vi "MakeHeaderFile.vi"(4 "Data File Name 2":path, 5 "Data File Name 1":path, 6 "Parameters":string, 7 "File Format":T1, 8 "error in (no error)":errorcluster, 9 "File Description":string, 10 "File Name":path, 11 "Date/Time sec (Now if empty)":dbl format="%.2f") -> (0 "error out":errorcluster, 1 "Complete text":string, 3 "Actual date/time":string)   [LabVIEW 2015]
uses:
  Controls/File formats.ctl
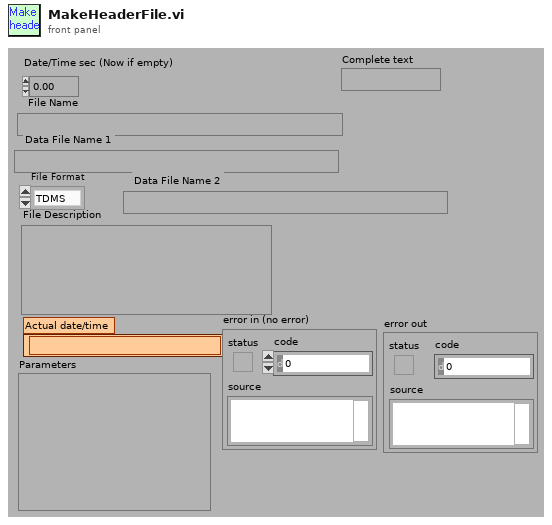
[diagram p1: front panel]
types:
  T1 = typedef "File formats.ctl" = enum16{"TDMS", "ASCII", "BINARY"}
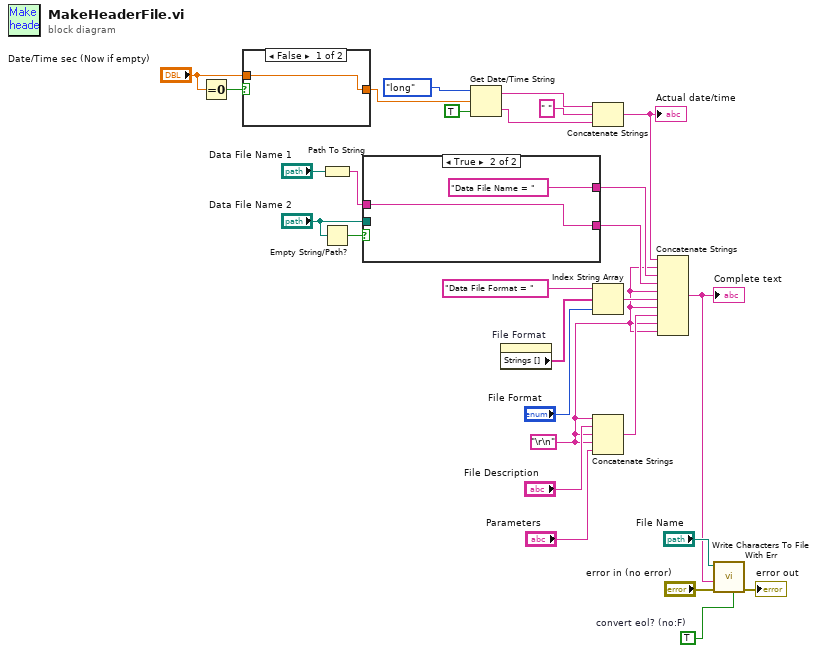
[diagram p0: block diagram]
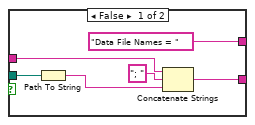
[diagram p2: hidden frame]
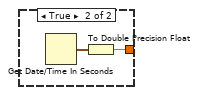
[diagram p3: hidden frame]
diagram:
  w25 = TRUE  # convert eol? (no:F)
  w3 = "\r\n"
  n1 = Equal To 0?(x="Date/Time sec (Now if empty)") -> (x = 0?=w18:bool)
  n2 = case shown="False" w18 {
    tunnel: [w29 w31] -> w24
    tunnel: "Date/Time sec (Now if empty)" -> [w29 _]
    frame False {
    }
    frame True {
      n3 = Get Date/Time In Seconds() -> (seconds since 1Jan1904=w30:timestamp)
      n4 = To Double Precision Float(number=w30) -> (double precision float=w31:dbl)
    }
  }
  n5 = Path To String(path="Data File Name 1") -> (string=w9:string)
  n6 = Empty String/Path?(string/path="Data File Name 2") -> (empty?=w8:bool)
  n7 = case shown="True" w8 {
    tunnel: w9 -> [w37 w39]
    tunnel: "Data File Name 2" -> [w36 _]
    tunnel: [w33 w39] -> w5
    tunnel: ["Data File Names = " ("Substring") "Data File Name = " ("Substring")] -> w6
    frame False {
      n8 = Path To String(path=w36) -> (string=w35:string)
      n9 = Concatenate Strings(w37, "; " ("Substring"), w35) -> (w33:string)
    }
    frame True {
    }
  }
  n10 = Get Date/Time String(date format (0)=enum16{"short", "long", "abbreviated"}."long", seconds (now)=w24, want seconds? (F)=TRUE) -> (date string=w22:string, time string=w21:string)
  n11 = property on="File Format" class="Enum (strict)"() -> ("Strings []"=w13:string[])  [unwired: 2 in, 2 out]
  n12 = Concatenate Strings(w22, " " ("time string"), w21) -> (w10:string)
  "Actual date/time" <- w10
  n13 = Index String Array(1:"File Format", 2:w13, 3:"Data File Format = " ("string (\"\")")) -> (0:w4:string)
  n14 = Concatenate Strings(w3, "File Description", w3, w3, "Parameters") -> (w26:string)
  n15 = Concatenate Strings(w10, w3, w6, w5, w3, w4, w3, w26, w3, w3) -> (w27:string)
  "Complete text" <- w27
  n16 = call "Write Characters To File With Err.vi"("convert eol? (no:F)"=w25, "error in (no error)"="error in (no error)", "character string"=w27, "file path (dialog if empty)"="File Name") -> ("error out"=→"error out":errorcluster)  [unwired: 1 in, 6 out]
